vi "Read DataSocket Configuration.vi"(8 "error in (no error)":errorcluster, 11 "DataSocket Client in":refnum<class "DataSocket Client.lvclass">) -> (0 "error out":errorcluster, 2 "Configuration":T1, 3 "DataSocket Client out":refnum<class "DataSocket Client.lvclass">)   [LabVIEW 2021, in "DataSocket Client.lvclass"]
uses:
  DataSocket Client.lvclass
  DataSocket Client.lvclass/DataSocket Client.ctl
  DataSocket Configuration.ctl
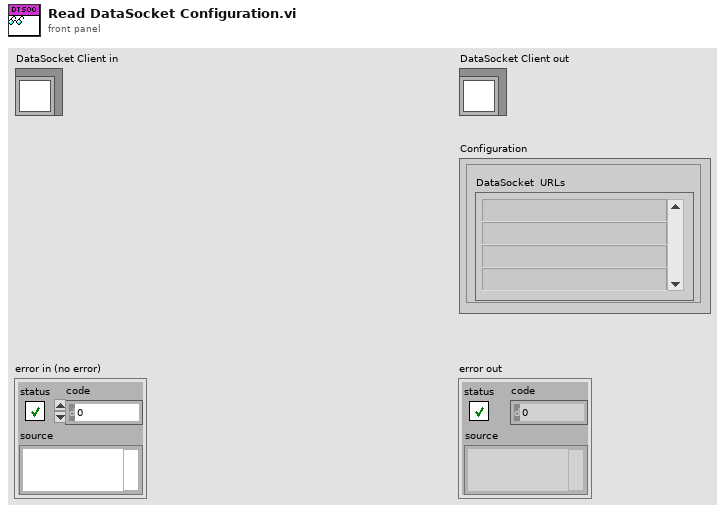
[diagram p1: front panel]
types:
  T1 = typedef "DataSocket Configuration.ctl" = cluster{"DataSocket  URLs":string[]}
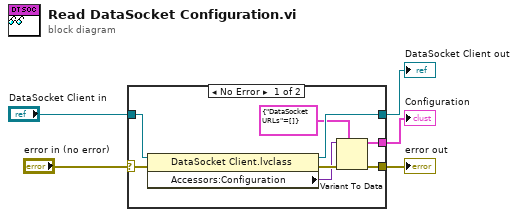
[diagram p0: block diagram]
diagram:
  n1 = case shown="No Error" "error in (no error)" {
    selector: "error in (no error)" -> [w13 w14]
    tunnel: [w12 w14] -> w4
    tunnel: [w9 w15] -> w2
    tunnel: "DataSocket Client in" -> [w10 w15]
    tunnel: [w6 _] -> w1
    frame No Error {
      n2 = property class="DataSocket Client.lvclass"(reference=w10, error in=w13) -> (reference out=w9:refnum<class "DataSocket Client.lvclass">, error out=w11:errorcluster, "Accessors:Configuration"=w8:variant)
      n3 = Variant To Data(error in=w11, type=T1 {"DataSocket  URLs"=[]} ("Configuration"), Variant=w8) -> (data=w6:T1, error out=w12:errorcluster)
    }
    frame Error {
    }
  }
  "error out" <- w4
  "DataSocket Client out" <- w2
  "Configuration" <- w1
